vi "NiFpga_HdlFifo_WriteU64.vi"(6 "timeout":u32, 7 "error in (no error)":errorcluster, 8 "data in":u64[](array[numeric]), 9 "fifo number":u32, 10 "fpga vi reference in":refnum<k20>) -> (0 "error out":errorcluster, 1 "empty elements remaining":u64, 3 "fpga vi reference out":refnum<k20>)   [LabVIEW 2023]
doc: "Dynamically reads the register at the provided offset. Set check for errors to true to check for errors such as if the register offset is invalid or if the register is running in an external clock domain that might not be running."
uses:
  NiFpga.dll
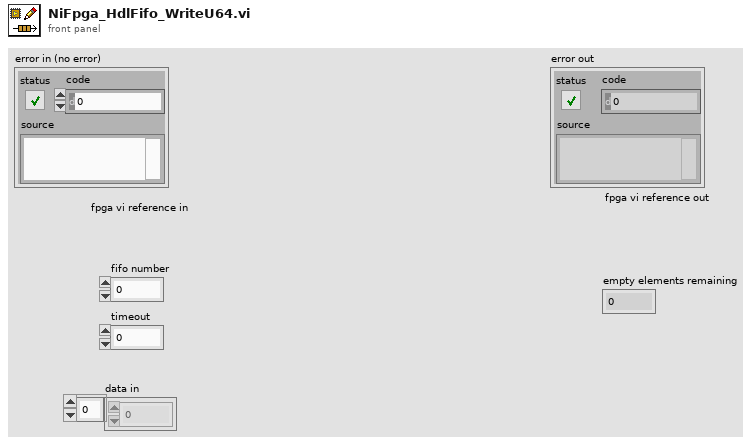
[diagram p1: front panel]
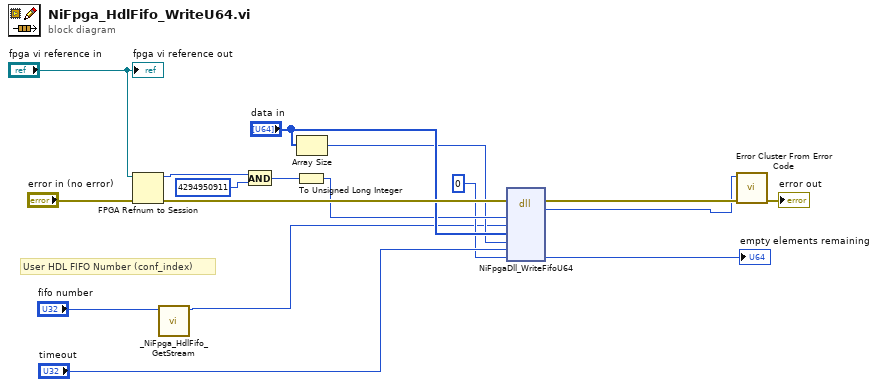
[diagram p0: block diagram]
diagram:
  # "User HDL FIFO Number (conf_index)"
  n1 = FPGA Refnum to Session(4:"error in (no error)", 7:"fpga vi reference in") -> (0:w12:errorcluster, 3:w14:u64)
  n2 = call "_NiFpga_HdlFifo_GetStream.vi"("Fifo Number"="fifo number") -> ("Fifo Stream"=w1:u32)  [unwired: 10 in]
  n3 = And(x=w14, y=u64 4294950911) -> (x .and. y?=w6:u64)
  n4 = To Unsigned Long Integer(number=w6) -> (unsigned 32bit integer=w5:u32)
  n5 = Array Size(array="data in") -> (size(s)=w4:i32)
  n6 = dll-call lib="NiFpga.*" fn="NiFpgaDll_WriteFifoU64"(error in=w12, "session"=w5, "fifo"=w1, "data"="data in", "numberOfElements"=w4, "timeout"="timeout", "emptyElementsRemainining"=u64 0) -> (error out=w11:errorcluster, "return type"=w10:i32, "emptyElementsRemainining"=→"empty elements remaining":u64)  [unwired: 7 in, 1 out]
  n7 = call <vilib>:"Error Cluster From Error Code.vi"("error in (no error)"=w11, "error code (0)"=w10) -> ("error out"=→"error out":errorcluster)  [unwired: 7 in]
  "fpga vi reference out" <- "fpga vi reference in"
